vi "Periodic Tasks.vi"(8 "error in":errorcluster) -> ()   [LabVIEW 2017]
doc: "This VI runs in parallel to other tasks. It can contain as many user-defined periodic loops as you need. These can carry out PID or other sorts of timed response."
uses:
  <vilib>/Rock Robotics/WPI/Solenoid/WPI_SolenoidValue.ctl
  <vilib>/Rock Robotics/WPI/ThirdParty/Phoenix-LabVIEW/Motor Controller/Controls/CTRE_Phoenix_MotorControl_ControlMode.ctl
  <vilib>/Rock Robotics/WPI/DriverStation/WPI_DriverStationRobotMode2.ctl
  LabVIEW_is_Under_Control.lib/Util/Toggle/Change Detect.vi
  LabVIEW_is_Under_Control.lib/Util/Toggle/Change Detect Boolean.vi
  Robot Global Data.vi
  <vilib>/Rock Robotics/WPI/Solenoid/WPI_SolenoidSetEnum.vi
panel:
  out "Yaw":dbl
  in  "Exchange":dbl
  in  "ScoringHigh":dbl
  in  "Scoring Low":dbl
  in  "Reset":bool
  in  "Gains Elevador":T1={"proportional gain (Kc)"=1.0, "integral time (Ti, min)"=0.01, "derivative time (Td, min)"=0.0} {"derivative time (Td, min)" format="%.3f"; "integral time (Ti, min)" format="%.3f"; "proportional gain (Kc)" format="%.3f"}
  in  "Range Elevador":cluster{"output high":dbl, "output low":dbl}={"output high"=0.6, "output low"=-0.6} {"output low" format="%.2f"; "output high" format="%.2f"}
  in  "Enable squared":bool
  in  "Score":dbl=-0.3
  in  "Segurando":dbl=0.3
  in  "Expelir":dbl=-0.3
  in  "Coletar":dbl=0.9
  # "Intake"
  # "Drivetrain"
  # "Elevador"
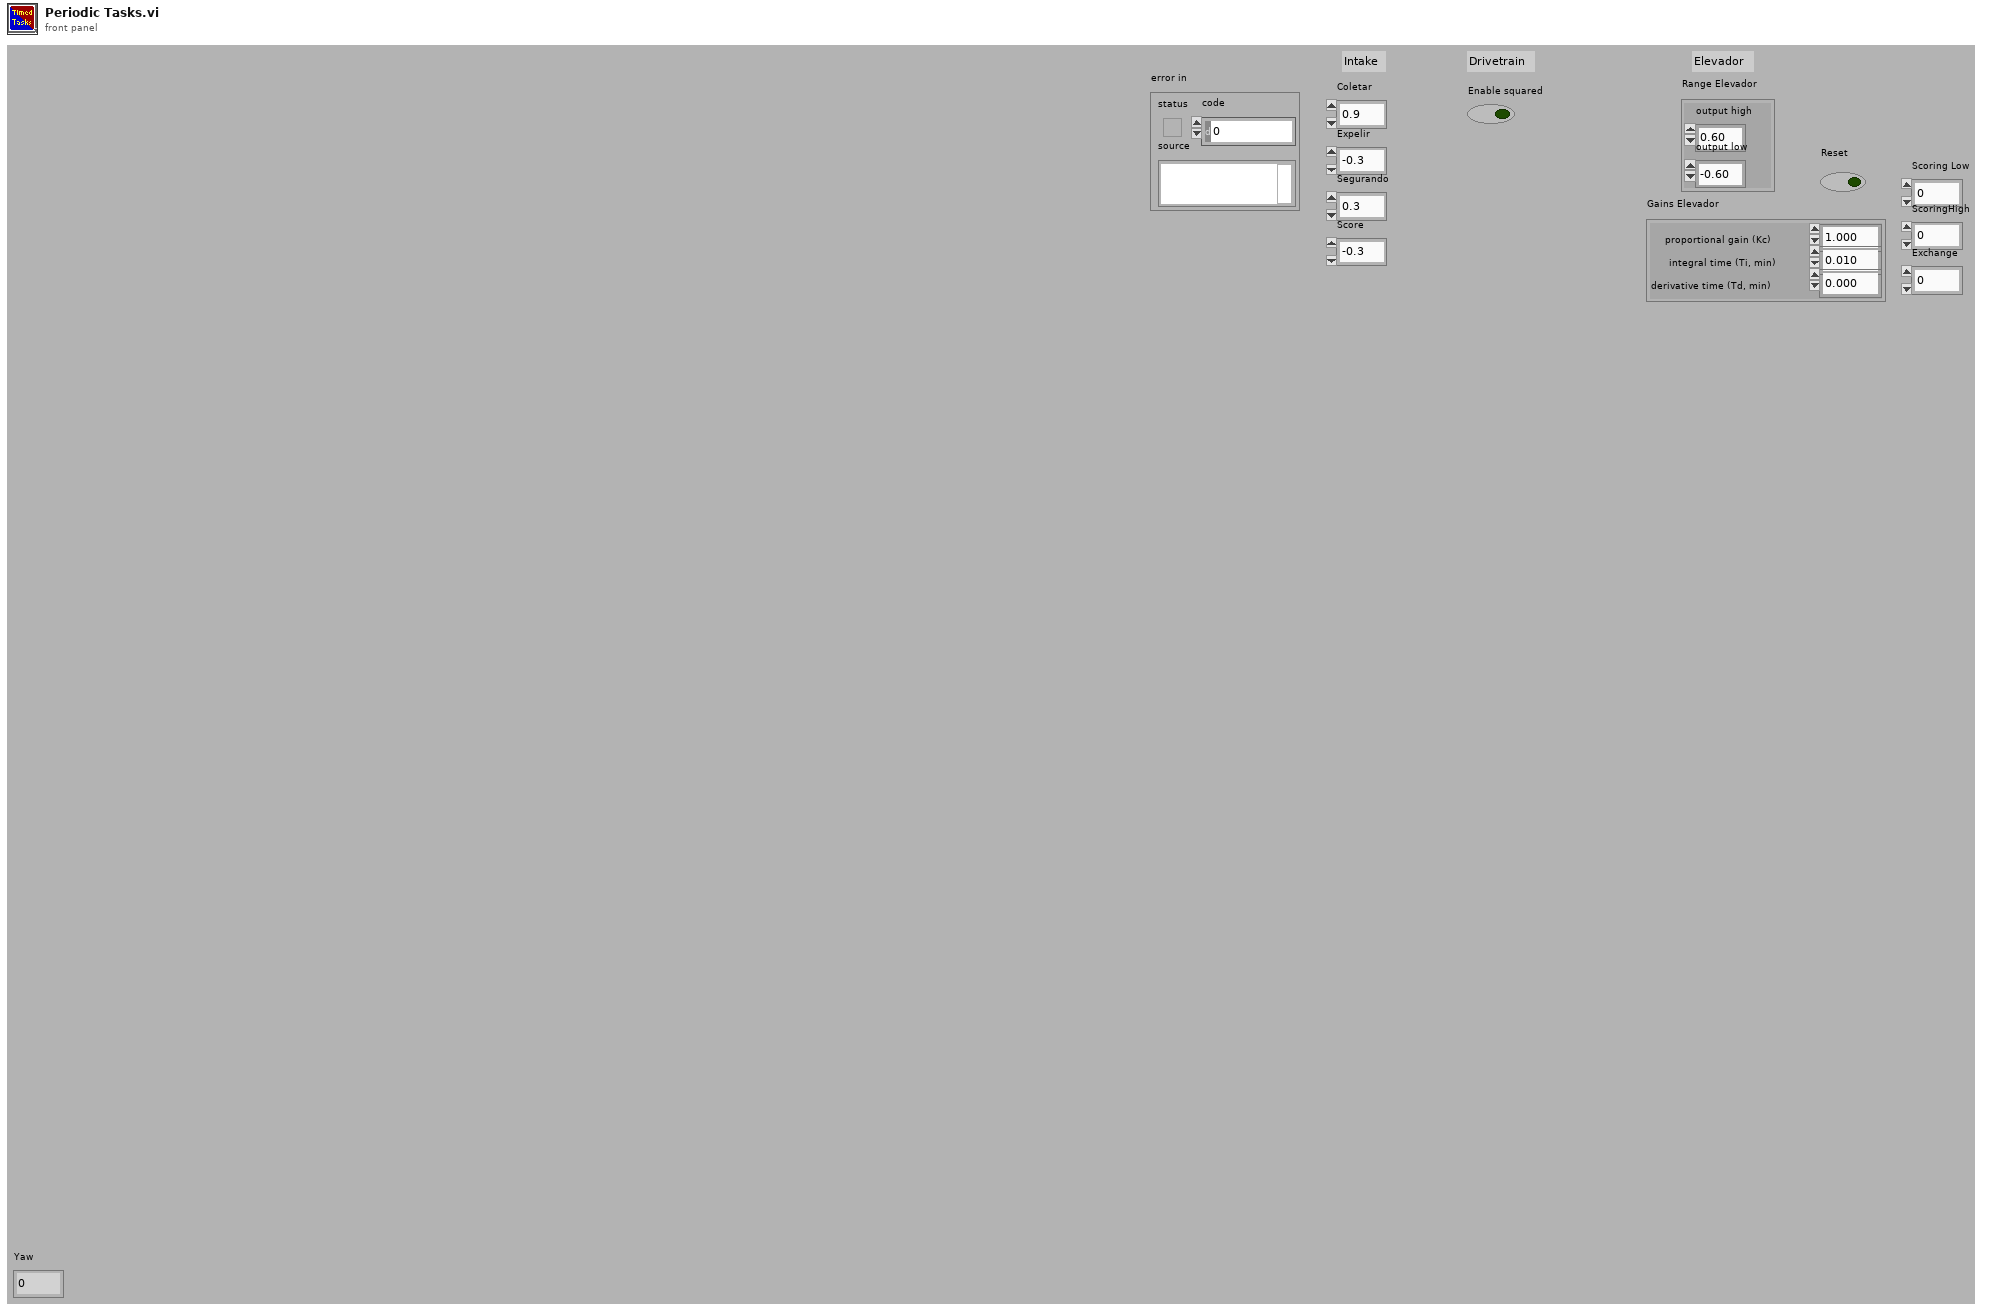
[diagram p1: front panel]
types:
  T1 = cluster{"proportional gain (Kc)":dbl, "integral time (Ti, min)":dbl, "derivative time (Td, min)":dbl}
  T2 = typedef "Máquina de estado do elevador.ctl" = enum16{"Resting", "Scoring Low", "Scoring Higher", "Exchange"}
  T3 = enum16{"Repouso", "Coletando", "Segurando", "Score"}
  T4 = typedef "WPI_SwitchDevRef.ctl" = cluster{"DevStatus":errorcluster, "DIO Channel":T5, "CntIndex":T6, "Normally Closed":bool}
  T5 = typedef "FPGA_DIOChannel.ctl" = enum8{"DIO 0", "DIO 1", "DIO 2", "DIO 3", "DIO 4", "DIO 5", "DIO 6", "DIO 7", "DIO 8", "DIO 9", "DIO MXP 0", "DIO MXP 1", "DIO MXP 2", "DIO MXP 3", "DIO MXP 4", "DIO MXP 5", "DIO MXP 6", "DIO MXP 7", "DIO MXP 8", "DIO MXP 9", "DIO MXP 10", "DIO MXP 11", "DIO MXP 12", "DIO MXP 13", "DIO MXP 14", "DIO MXP 15", "SPI Port CS1", "SPI Port CS2", "SPI Port CS3", "SPI Port MISO", "SPI Port MOSI", "Invalid"}
  T6 = typedef "FPGA_CounterCtrSystemIndex.ctl" = enum8{"Ctr 0", "Ctr 1", "Ctr 2", "Ctr 3", "Ctr 4", "Ctr 5", "Ctr 6", "Ctr 7", "Invalid"}
  T7 = typedef "WPI_EncoderDevRef.ctl" = cluster{"DevStatus":errorcluster, "EncoderIndex":T8, "CounterIndex":T6, "DistancePerCount":dbl, "Decoding Type":T9}
  T8 = typedef "FPGA_EncoderIdx.ctl" = enum8{"Enc 0", "Enc 1", "Enc 2", "Enc 3", "Enc 4", "Enc 5", "Enc 6", "Enc 7", "Invalid"}
  T9 = typedef "WPI_EncoderType.ctl" = enum16{"1x", "2x", "4x"}
  T10 = typedef "WPI_SolenoidDevRef.ctl" = cluster{"DevStatus":errorcluster, "Pneumatics Control Module":u8, "Forward Solenoid Channel":T11, "Reverse Solenoid Channel":T11}
  T11 = typedef "WPI_SolenoidChannel.ctl" = enum8{"Solenoid 0", "Solenoid 1", "Solenoid 2", "Solenoid 3", "Solenoid 4", "Solenoid 5", "Solenoid 6", "Solenoid 7", "Invalid"}
  T12 = typedef "WPI_MotorControlDeviceRef.ctl" = cluster{"DeviceStatus":errorcluster, "Type":T13, "PWM":cluster{"PWM Channel":T14, "DeadBand":T15}, "CAN":cluster{"Device Number":u8, "SetOutput VI Ref":variant, "GetOutput VI Ref":variant, "Enable VI Ref":variant, "Disable VI Ref":variant, "Data":variant}, "Invert":bool, "DIO PWM":cluster{"PWM \"Enable\" Channel":T14, "DIOChannel":T5, "PWM Rate":dbl}}
  T13 = typedef "WPI_MotorControlType.ctl" = enum16{"PWM", "CAN", "DIO PWM"}
  T14 = typedef "FPGA_DIOPWMChannel.ctl" = enum8{"PWM 0", "PWM 1", "PWM 2", "PWM 3", "PWM 4", "PWM 5", "PWM 6", "PWM 7", "PWM 8", "PWM 9", "PWM MXP 0", "PWM MXP 1", "PWM MXP 2", "PWM MXP 3", "PWM MXP 4", "PWM MXP 5", "PWM MXP 6", "PWM MXP 7", "PWM MXP 8", "PWM MXP 9", "Invalid"}
  T15 = typedef "WPI_PWMDeadband.ctl" = cluster{"Name":string, "maxPositivePwm":i32, "minPositivePwm":i32, "centerPwm":i32, "maxNegativePwm":i32, "minNegativePwm":i32, "angularRange":u16}
  T16 = cluster{"Yaw":dbl, "Roll":dbl, "Pitch":dbl, "Heading":dbl, "Fused Heading":dbl}
  T17 = typedef "WPI_SolenoidValue.ctl" = enum16{"Off", "On", "Forward", "Reverse"}
  T18 = typedef "WPI_DriverStationRobotMode2.ctl" = enum16{"Autonomous Disabled", "Autonomous Enabled", "Teleop Disabled", "Teleop Enabled", "Disconnected", "Finish", "Test Disabled", "Test Enabled", "Emergency Stopped"}
  T19 = typedef "CTRE_Phoenix_MotorControl_ControlMode.ctl" = u16
  T20 = typedef "Axes Cluster.ctl" = cluster{"Axes[0]":dbl, "Axes[1]":dbl, "Axes[2]":dbl, "Axes[3]":dbl, "Axes[4]":dbl, "Axes[5]":dbl, "Axes[6]":dbl, "Axes[7]":dbl, "Axes[8]":dbl}
  T21 = typedef "Button Cluster.ctl" = cluster{"Buttons[0]":bool, "Buttons[1]":bool, "Buttons[2]":bool, "Buttons[3]":bool, "Buttons[4]":bool, "Buttons[5]":bool, "Buttons[6]":bool, "Buttons[7]":bool, "Buttons[8]":bool, "Buttons[9]":bool}
  T22 = typedef "D-Pad.ctl" = cluster{"Top":bool, "Bottom":bool, "None":bool, "Right":bool, "Left":bool}
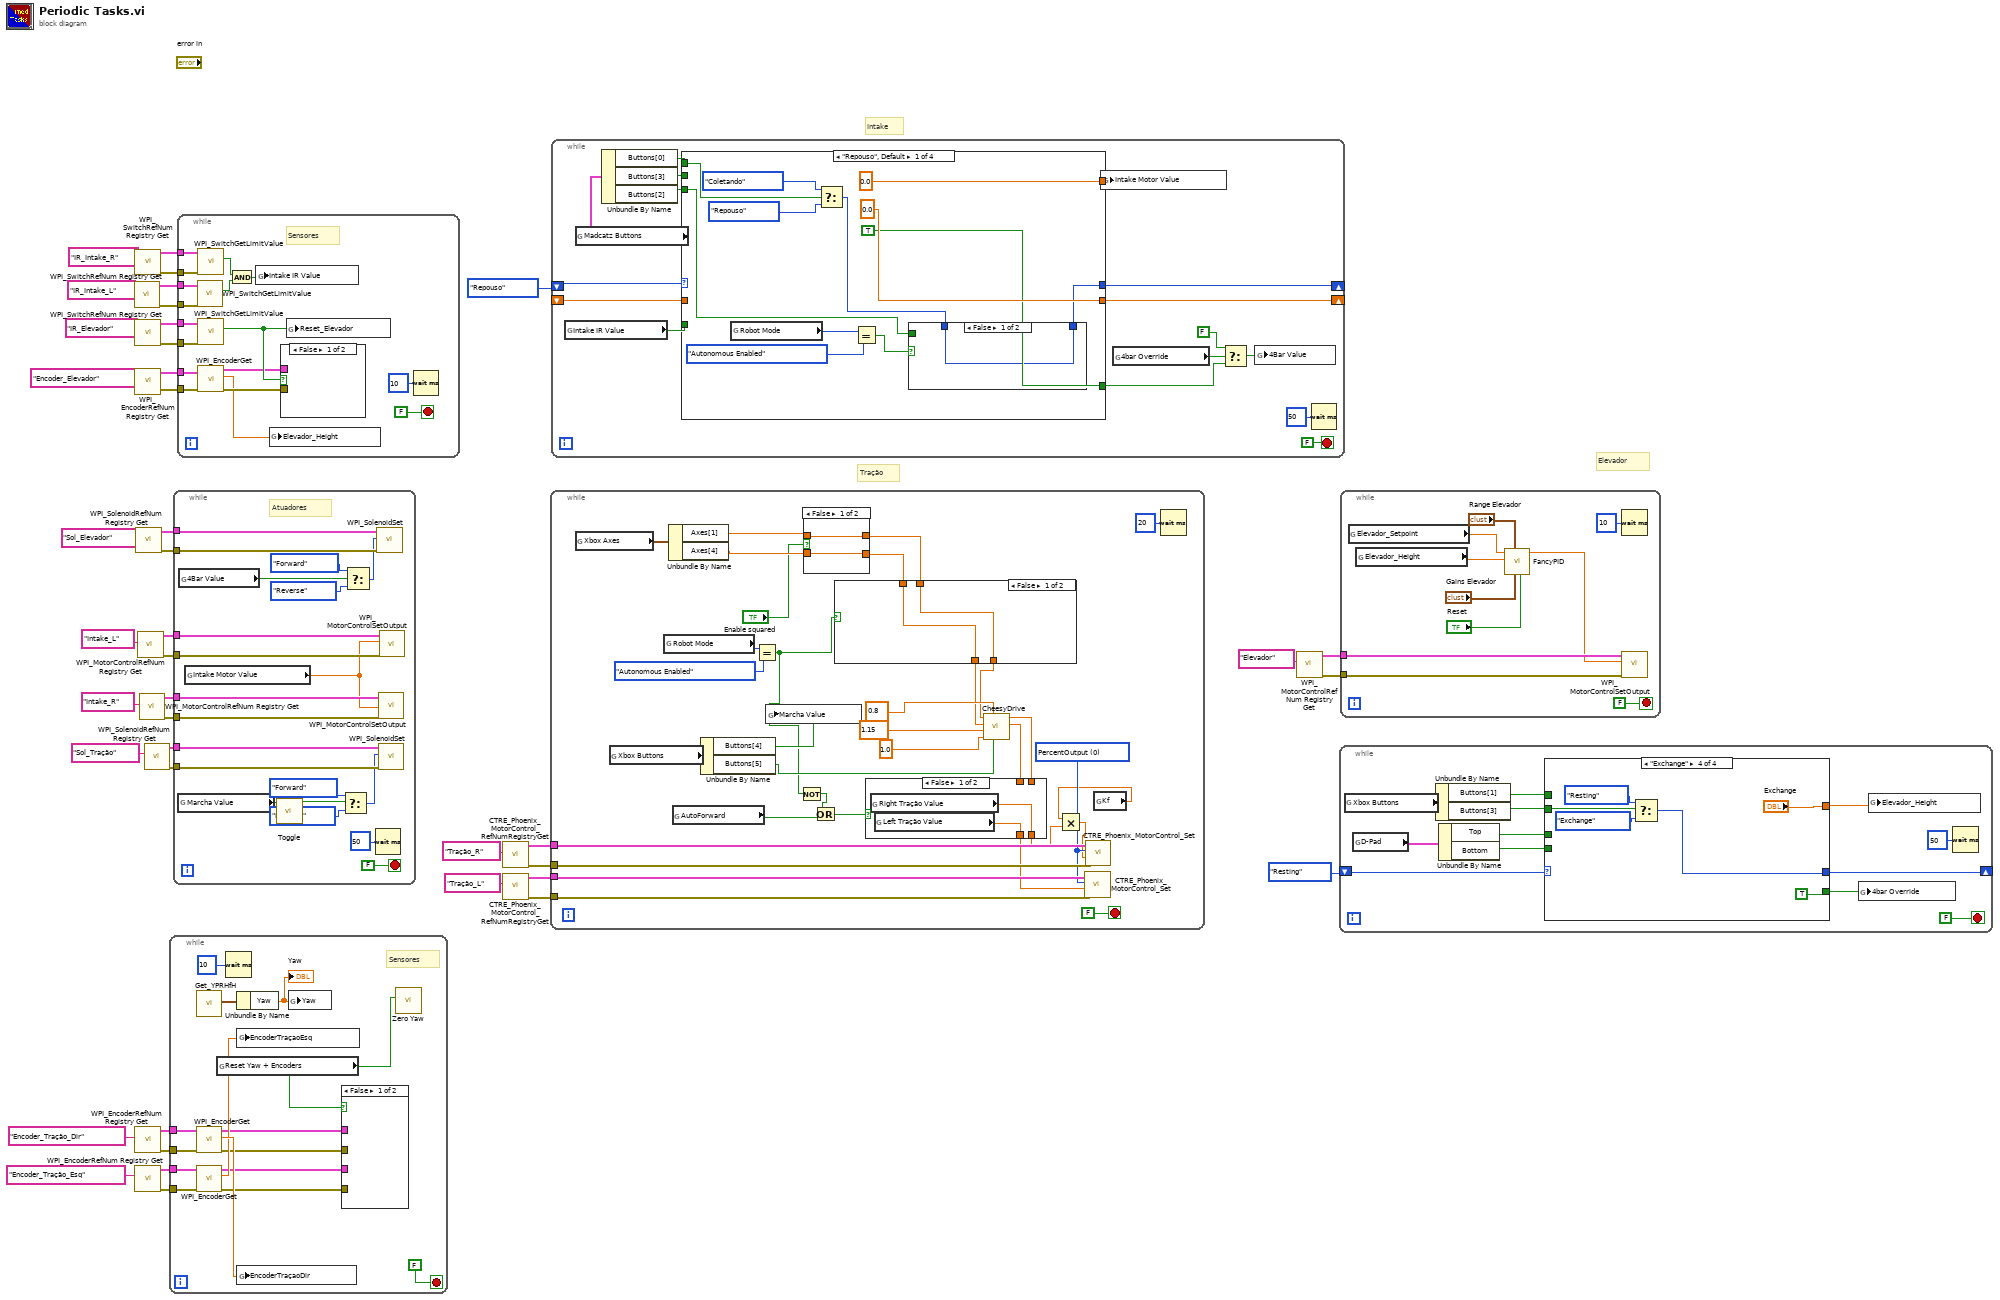
[diagram p0: block diagram]
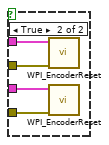
[diagram p2: hidden frame]
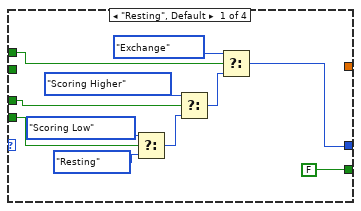
[diagram p3: hidden frame]
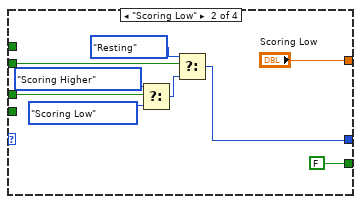
[diagram p4: hidden frame]
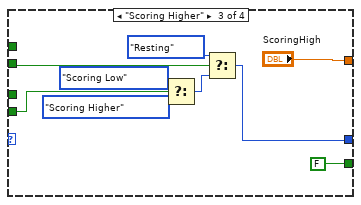
[diagram p5: hidden frame]
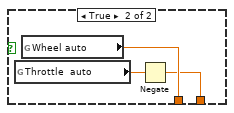
[diagram p7: hidden frame]
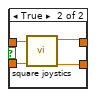
[diagram p8: hidden frame]
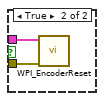
[diagram p9: hidden frame]
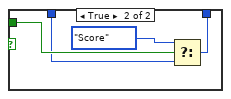
[diagram p10: hidden frame]
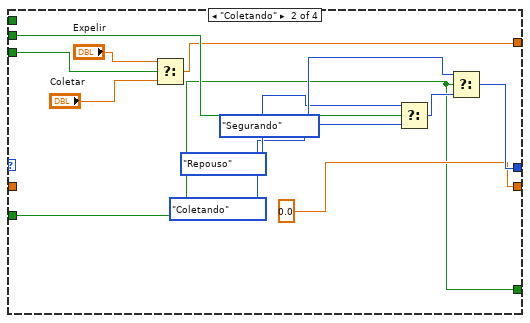
[diagram p11: hidden frame]
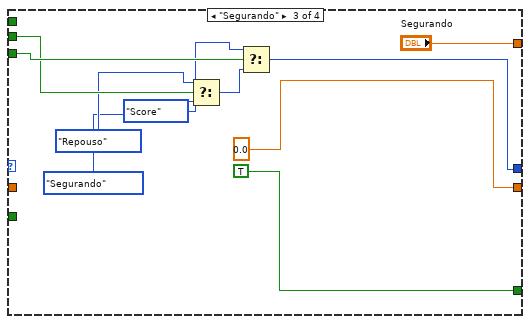
[diagram p12: hidden frame]
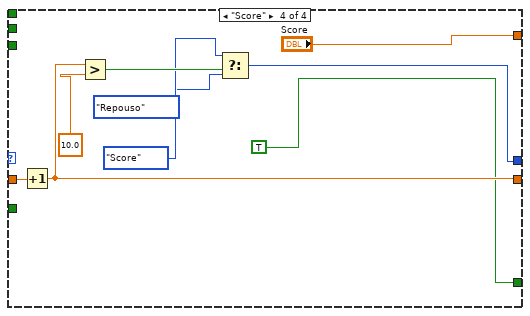
[diagram p13: hidden frame]
diagram:
  # "Elevador"
  # "Tração"
  # "Intake"
  n1 = call <vilib>:"WPI_SwitchRefNum Registry Get.vi"("refnum name"="IR_Intake_L") -> ("error out"=w38:errorcluster, "SwitchDevRef"=w37:T4)  [unwired: 9 in]
  n2 = call <vilib>:"WPI_SwitchRefNum Registry Get.vi"("refnum name"="IR_Intake_R") -> ("error out"=w36:errorcluster, "SwitchDevRef"=w35:T4)  [unwired: 9 in]
  n3 = call <vilib>:"WPI_SwitchRefNum Registry Get.vi"("refnum name"="IR_Elevador") -> ("error out"=w15:errorcluster, "SwitchDevRef"=w16:T4)  [unwired: 9 in]
  n4 = call <vilib>:"WPI_EncoderRefNum Registry Get.vi"("refnum name"="Encoder_Elevador") -> ("error out"=w11:errorcluster, "EncoderDevRef"=w12:T7)  [unwired: 9 in]
  n5 = call <vilib>:"WPI_EncoderRefNum Registry Get.vi"("refnum name"="Encoder_Tração_Dir") -> ("error out"=w4:errorcluster, "EncoderDevRef"=w5:T7)  [unwired: 9 in]
  n6 = call <vilib>:"WPI_EncoderRefNum Registry Get.vi"("refnum name"="Encoder_Tração_Esq") -> ("error out"=w3:errorcluster, "EncoderDevRef"=w2:T7)  [unwired: 9 in]
  n7 = call <vilib>:"WPI_SolenoidRefNum Registry Get.vi"("refnum name"="Sol_Elevador") -> ("error out"=w33:errorcluster, "SolenoidDevRef"=w32:T10)  [unwired: 9 in]
  n8 = call <vilib>:"WPI_MotorControlRefNum Registry Get.vi"("refnum name"="Intake_L") -> ("error out"=w31:errorcluster, "MotorControlDevRef"=w30:T12)  [unwired: 9 in]
  n9 = call <vilib>:"WPI_MotorControlRefNum Registry Get.vi"("refnum name"="Intake_R") -> ("error out"=w26:errorcluster, "MotorControlDevRef"=w27:T12)  [unwired: 9 in]
  n10 = call <vilib>:"WPI_SolenoidRefNum Registry Get.vi"("refnum name"="Sol_Tração") -> ("error out"=w23:errorcluster, "SolenoidDevRef"=w24:T10)  [unwired: 9 in]
  n11 = while {
    tunnel: w5 -> [w56]
    tunnel: w4 -> [w55]
    tunnel: w2 -> [w51]
    tunnel: w3 -> [w52]
    stop <- FALSE stop-if-true
    # "Sensores"
    n12 = call <vilib>:"Get_YPRHfH.vi"() -> ("YRPHfH"=w44:T16)  [unwired: 11 in]
    n13 = call <vilib>:"WPI_EncoderGet.vi"("error in (no error)"=w55, "EncoderDevRef"=w56) -> ("error out"=w47:errorcluster, "Distance"=w54:dbl, "EncoderDevRef"=w48:T7)  [unwired: 4 in, 3 out]
    n14 = call <vilib>:"WPI_EncoderGet.vi"("error in (no error)"=w52, "EncoderDevRef"=w51) -> ("error out"=w45:errorcluster, "Distance"=w53:dbl, "EncoderDevRef"=w46:T7)  [unwired: 4 in, 3 out]
    n15 = global read "Robot Global Data.vi" "Reset Yaw + Encoders"() -> (w42:bool)
    n16 = Wait (ms)(milliseconds to wait=u32 10) -> ()  [unwired: 1 out]
    n17 = Unbundle By Name(w44) -> ("Yaw"=w43:dbl)
    "Yaw" <- w43
    n18 = global write "Robot Global Data.vi" "EncoderTraçaoEsq"(w53) -> ()
    n19 = global write "Robot Global Data.vi" "EncoderTraçaoDir"(w54) -> ()
    n20 = global write "Robot Global Data.vi" "Yaw"(w43) -> ()
    n21 = case shown="False" w42 {
      tunnel: w48 -> [_ w60]
      tunnel: w47 -> [_ w59]
      tunnel: w46 -> [_ w58]
      tunnel: w45 -> [_ w57]
      frame False {
      }
      frame True {
        n22 = call <vilib>:"WPI_EncoderReset.vi"("error in (no error)"=w59, "EncoderDevRef"=w60) -> ()  [unwired: 8 in, 2 out]
        n23 = call <vilib>:"WPI_EncoderReset.vi"("error in (no error)"=w57, "EncoderDevRef"=w58) -> ()  [unwired: 8 in, 2 out]
      }
    }
    n24 = call <vilib>:"Zero Yaw.vi"("Zero"=w42) -> ()  [unwired: 11 in]
  }
  n25 = while {
    tunnel: w33 -> [w80]
    tunnel: w32 -> [w79]
    tunnel: w31 -> [w74]
    tunnel: w30 -> [w73]
    tunnel: w27 -> [w72]
    tunnel: w26 -> [w71]
    tunnel: w24 -> [w65]
    tunnel: w23 -> [w64]
    stop <- FALSE stop-if-true
    # "Atuadores"
    n26 = global read "Robot Global Data.vi" "Marcha Value"() -> (w62:bool)
    n27 = global read "Robot Global Data.vi" "4Bar Value"() -> (w75:bool)
    n28 = global read "Robot Global Data.vi" "Intake Motor Value"() -> (w70:dbl)
    n29 = call "Toggle.vi"("In"=w62) -> ("Toggled"=w61:bool)  [unwired: 10 in]
    n30 = Select(t=WPI_SolenoidValue."Forward" ("Value"), s=w61, f=WPI_SolenoidValue."Reverse" ("Value")) -> (s? t:f=w63:T17)
    n31 = Select(t=WPI_SolenoidValue."Forward" ("Value"), s=w75, f=WPI_SolenoidValue."Reverse" ("Value")) -> (s? t:f=w78:T17)
    n32 = Wait (ms)(milliseconds to wait=u32 50) -> ()  [unwired: 1 out]
    n33 = call-poly <vilib>:"WPI_SolenoidSet.vi"("error in (no error)"=w80, "Value"=w78, "SolenoidDevRef"=w79) -> ()  [unwired: 7 in, 2 out]
    n34 = call <vilib>:"WPI_MotorControlSetOutput.vi"("error in (no error)"=w71, "Output"=w70, "MotorControlDevRef"=w72) -> ()  [unwired: 6 in, 3 out]
    n35 = call-poly <vilib>:"WPI_SolenoidSet.vi"("error in (no error)"=w64, "Value"=w63, "SolenoidDevRef"=w65) -> ()  [unwired: 7 in, 2 out]
    n36 = call <vilib>:"WPI_MotorControlSetOutput.vi"("error in (no error)"=w74, "Output"=w70, "MotorControlDevRef"=w73) -> ()  [unwired: 6 in, 3 out]
  }
  n37 = while {
    tunnel: w38 -> [w92]
    tunnel: w37 -> [w91]
    tunnel: w36 -> [w90]
    tunnel: w35 -> [w89]
    tunnel: w15 -> [w87]
    tunnel: w16 -> [w88]
    tunnel: w12 -> [w86]
    tunnel: w11 -> [w85]
    stop <- FALSE stop-if-true
    # "Sensores"
    n38 = call <vilib>:"WPI_SwitchGetLimitValue.vi"("error in (no error)"=w92, "SwitchDevRef"=w91) -> ("Switch Pressed"=w97:bool)  [unwired: 7 in, 2 out]
    n39 = call <vilib>:"WPI_SwitchGetLimitValue.vi"("error in (no error)"=w90, "SwitchDevRef"=w89) -> ("Switch Pressed"=w96:bool)  [unwired: 7 in, 2 out]
    n40 = call <vilib>:"WPI_SwitchGetLimitValue.vi"("error in (no error)"=w87, "SwitchDevRef"=w88) -> ("Switch Pressed"=w84:bool)  [unwired: 7 in, 2 out]
    n41 = call <vilib>:"WPI_EncoderGet.vi"("error in (no error)"=w85, "EncoderDevRef"=w86) -> ("error out"=w82:errorcluster, "Distance"=w81:dbl, "EncoderDevRef"=w83:T7)  [unwired: 4 in, 3 out]
    n42 = And(x=w96, y=w97) -> (x .and. y?=w93:bool)
    n43 = global write "Robot Global Data.vi" "Intake IR Value"(w93) -> ()
    n44 = global write "Robot Global Data.vi" "Elevador_Height"(w81) -> ()
    n45 = case shown="False" w84 {
      tunnel: w83 -> [_ w99]
      tunnel: w82 -> [_ w98]
      frame False {
      }
      frame True {
        n46 = call <vilib>:"WPI_EncoderReset.vi"("error in (no error)"=w98, "EncoderDevRef"=w99) -> ()  [unwired: 8 in, 2 out]
      }
    }
    n47 = global write "Robot Global Data.vi" "Reset_Elevador"(w84) -> ()
    n48 = Wait (ms)(milliseconds to wait=u32 10) -> ()  [unwired: 1 out]
  }
  n49 = call <vilib>:"CTRE_Phoenix_MotorControl_RefNumRegistryGet.vi"("refnum name"="Tração_R") -> ("error out"=w18:errorcluster, "PhoenixMotorControlDevRef"=w20:T12)  [unwired: 9 in]
  n50 = call <vilib>:"CTRE_Phoenix_MotorControl_RefNumRegistryGet.vi"("refnum name"="Tração_L") -> ("error out"=w17:errorcluster, "PhoenixMotorControlDevRef"=w19:T12)  [unwired: 9 in]
  n51 = while {
    tunnel: w20 -> [w123]
    tunnel: w19 -> [w122]
    tunnel: w18 -> [w121]
    tunnel: w17 -> [w120]
    stop <- FALSE stop-if-true
    w119 = T19 0 items=["PercentOutput"=0, "Position"=1, "Velocity"=2, "Current"=3, "Follower"=5, "MotionProfile"=6, "MotionMagic"=7, "MotionMagicArc"=8, "MotionProfileArc"=10, "Disabled"=15] ("Control Mode")
    n52 = global read "Robot Global Data.vi" "Xbox Axes"() -> (w132:T20)
    n53 = global read "Robot Global Data.vi" "Xbox Buttons"() -> (w130:T21)
    n54 = global read "Robot Global Data.vi" "Robot Mode"() -> (w115:T18)
    n55 = Unbundle By Name(w132) -> ("Axes[1]"=w117:dbl, "Axes[4]"=w118:dbl)
    n56 = global read "Robot Global Data.vi" "AutoForward"() -> (w104:bool)
    n57 = Unbundle By Name(w130) -> ("Buttons[4]"=w128:bool, "Buttons[5]"=w129:bool)
    n58 = Equal?(x=w115, y=WPI_DriverStationRobotMode2."Autonomous Enabled") -> (x = y?=w103:bool)
    n59 = global write "Robot Global Data.vi" "Marcha Value"(w128) -> ()
    n60 = Not(x=w103) -> (.not. x?=w106:bool)
    n61 = case shown="False" "Enable squared" {
      tunnel: w118 -> [w143 w147]
      tunnel: [w143 w146] -> w112
      tunnel: w117 -> [w142 w145]
      tunnel: [w142 w144] -> w113
      frame False {
      }
      frame True {
        n62 = call "square joystics.vi"("right joy"=w147, "left joy"=w145) -> ("Right Out"=w146:dbl, "Left Out"=w144:dbl)  [unwired: 8 in]
      }
    }
    n63 = Or(x=w106, y=w104) -> (x .or. y?=w105:bool)
    n64 = case shown="False" w103 {
      tunnel: [w137 w141] -> w107
      tunnel: [w138 w139] -> w108
      tunnel: w113 -> [w138 _]
      tunnel: w112 -> [w137 _]
      frame False {
      }
      frame True {
        n65 = global read "Robot Global Data.vi" "Throttle  auto"() -> (w140:dbl)
        n66 = global read "Robot Global Data.vi" "Wheel auto"() -> (w141:dbl)
        n67 = Negate(x=w140) -> (-x=w139:dbl)
      }
    }
    n68 = call "CheesyDrive.vi"("Quickturn"=w129, "WheelNonLinearity"=0.8, "negInertiaScalar"=1.0, "Sensitivty"=1.15, "Wheel"=w107, "Throttle"=w108) -> ("Right PWM"=w109:dbl, "Left PWM"=w111:dbl)  [unwired: 4 in]
    n69 = case shown="False" w105 {
      tunnel: [w133 w135] -> w102
      tunnel: w111 -> [_ w135]
      tunnel: [w134 w136] -> w110
      tunnel: w109 -> [_ w136]
      frame False {
        n70 = global read "Robot Global Data.vi" "Right Tração Value"() -> (w133:dbl)
        n71 = global read "Robot Global Data.vi" "Left Tração Value"() -> (w134:dbl)
      }
      frame True {
      }
    }
    n72 = call <vilib>:"CTRE_Phoenix_MotorControl_Set.vi"("error in (no error)"=w120, "Output"=w110, "Control Mode"=w119, "PhoenixMotorControlDevRef"=w122) -> ()  [unwired: 6 in, 2 out]
    n73 = global read "Robot Global Data.vi" "Kf"() -> (w101:dbl)
    n74 = Multiply(x=w101, y=w102) -> (x*y=w100:dbl)
    n75 = call <vilib>:"CTRE_Phoenix_MotorControl_Set.vi"("error in (no error)"=w121, "Output"=w100, "Control Mode"=w119, "PhoenixMotorControlDevRef"=w123) -> ()  [unwired: 6 in, 2 out]
    n76 = Wait (ms)(milliseconds to wait=u32 20) -> ()  [unwired: 1 out]
  }
  n77 = while {
    shift-right: [w159] -> _
    shift-left: T3."Repouso" -> [w163]
    shift-right: [w156] -> _
    shift-left: _ -> [w157]
    stop <- FALSE stop-if-true
    n78 = global read "Robot Global Data.vi" "Intake IR Value"() -> (w158:bool)
    n79 = global read "Robot Global Data.vi" "Madcatz Buttons"() -> (w160:T21)
    n80 = Unbundle By Name(w160) -> ("Buttons[0]"=w152:bool, "Buttons[3]"=w154:bool, "Buttons[2]"=w153:bool)
    n81 = case shown="\"Repouso\", Default" w163 {
      tunnel: w152 -> [w175 _ _ _]
      tunnel: [w165 w188 w196 w205] -> w159
      tunnel: w154 -> [_ w191 w200 _]
      tunnel: w158 -> [_ w182 _ _]
      tunnel: w153 -> [w164 w181 w202 _]
      tunnel: w157 -> [_ _ _ w211]
      tunnel: [0.0 0.0 0.0 w210] -> w156
      tunnel: [0.0 w183 "Segurando" "Score"] -> w155
      tunnel: [TRUE w182 TRUE TRUE] -> w150
      frame "Repouso", Default {
        n82 = global read "Robot Global Data.vi" "Robot Mode"() -> (w168:T18)
        n83 = Select(t=T3."Coletando", s=w175, f=T3."Repouso") -> (s? t:f=w166:T3)
        n84 = Equal?(x=w168, y=WPI_DriverStationRobotMode2."Autonomous Enabled") -> (x = y?=w167:bool)
        n85 = case shown="False" w167 {
          tunnel: w164 -> [_ w180]
          tunnel: w166 -> [w176 w179]
          tunnel: [w176 w177] -> w165
          frame False {
          }
          frame True {
            n86 = Select(t=T3."Score", s=w180, f=w179) -> (s? t:f=w177:T3)
          }
        }
      }
      frame "Coletando" {
        n87 = Select(t="Expelir", s=w181, f="Coletar") -> (s? t:f=w183:dbl)
        n88 = Select(t=T3."Repouso", s=w191, f=T3."Coletando") -> (s? t:f=w185:T3)
        n89 = Select(t=T3."Segurando", s=w182, f=w185) -> (s? t:f=w188:T3)
      }
      frame "Segurando" {
        n90 = Select(t=T3."Repouso", s=w200, f=T3."Segurando") -> (s? t:f=w199:T3)
        n91 = Select(t=T3."Score", s=w202, f=w199) -> (s? t:f=w196:T3)
      }
      frame "Score" {
        n92 = Increment(x=w211) -> (x+1=w210:dbl)
        n93 = Greater?(x=w210, y=10.0) -> (0:w208:bool)
        n94 = Select(t=T3."Repouso", s=w208, f=T3."Score") -> (s? t:f=w205:T3)
      }
    }
    n95 = global write "Robot Global Data.vi" "Intake Motor Value"(w155) -> ()
    n96 = global read "Robot Global Data.vi" "4bar Override"() -> (w151:bool)
    n97 = Select(t=FALSE, s=w151, f=w150) -> (s? t:f=w148:bool)
    n98 = global write "Robot Global Data.vi" "4Bar Value"(w148) -> ()
    n99 = Wait (ms)(milliseconds to wait=u32 50) -> ()  [unwired: 1 out]
  }
  n100 = call <vilib>:"WPI_MotorControlRefNum Registry Get.vi"("refnum name"="Elevador") -> ("error out"=w8:errorcluster, "MotorControlDevRef"=w9:T12)  [unwired: 9 in]
  n101 = while {
    shift-right: [w213] -> _
    shift-left: Máquina_de_estado_do_elevador."Resting" -> [w214]
    stop <- FALSE stop-if-true
    n102 = global read "Robot Global Data.vi" "Xbox Buttons"() -> (w220:T21)
    n103 = global read "Robot Global Data.vi" "D-Pad"() -> (w221:T22)
    n104 = Unbundle By Name(w220) -> ("Buttons[1]"=w215:bool, "Buttons[3]"=w219:bool)
    n105 = Unbundle By Name(w221) -> ("Top"=w218:bool, "Bottom"=w217:bool)
    n106 = case shown="\"Exchange\"" w214 {
      tunnel: w219 -> [_ w242 w251 w257]
      tunnel: w218 -> [w233 w241 _ _]
      tunnel: w217 -> [w232 _ w249 _]
      tunnel: [_ "Scoring Low" "ScoringHigh" "Exchange"] -> w216
      tunnel: [w225 w239 w248 w256] -> w213
      tunnel: w215 -> [w230 _ _ _]
      tunnel: [FALSE FALSE FALSE TRUE] -> w212
      frame "Resting", Default {
        n107 = Select(t=Máquina_de_estado_do_elevador."Scoring Low", s=w232, f=Máquina_de_estado_do_elevador."Resting") -> (s? t:f=w234:T2)
        n108 = Select(t=Máquina_de_estado_do_elevador."Scoring Higher", s=w233, f=w234) -> (s? t:f=w231:T2)
        n109 = Select(t=Máquina_de_estado_do_elevador."Exchange", s=w230, f=w231) -> (s? t:f=w225:T2)
      }
      frame "Scoring Low" {
        n110 = Select(t=Máquina_de_estado_do_elevador."Scoring Higher", s=w241, f=Máquina_de_estado_do_elevador."Scoring Low") -> (s? t:f=w240:T2)
        n111 = Select(t=Máquina_de_estado_do_elevador."Resting", s=w242, f=w240) -> (s? t:f=w239:T2)
      }
      frame "Scoring Higher" {
        n112 = Select(t=Máquina_de_estado_do_elevador."Scoring Low", s=w249, f=Máquina_de_estado_do_elevador."Scoring Higher") -> (s? t:f=w250:T2)
        n113 = Select(t=Máquina_de_estado_do_elevador."Resting", s=w251, f=w250) -> (s? t:f=w248:T2)
      }
      frame "Exchange" {
        n114 = Select(t=Máquina_de_estado_do_elevador."Resting", s=w257, f=Máquina_de_estado_do_elevador."Exchange") -> (s? t:f=w256:T2)
      }
    }
    n115 = global write "Robot Global Data.vi" "4bar Override"(w212) -> ()
    n116 = global write "Robot Global Data.vi" "Elevador_Height"(w216) -> ()
    n117 = Wait (ms)(milliseconds to wait=u32 50) -> ()  [unwired: 1 out]
  }
  n118 = while {
    tunnel: w9 -> [w266]
    tunnel: w8 -> [w265]
    stop <- FALSE stop-if-true
    n119 = global read "Robot Global Data.vi" "Elevador_Setpoint"() -> (w260:dbl)
    n120 = global read "Robot Global Data.vi" "Elevador_Height"() -> (w259:dbl)
    n121 = call "FancyPID.vi"("Reset"="Reset", "Gains"="Gains Elevador", "Range"="Range Elevador", "Process variable"=w259, "Setpoint"=w260) -> ("output"=w264:dbl)  [unwired: 6 in]
    n122 = Wait (ms)(milliseconds to wait=u32 10) -> ()  [unwired: 1 out]
    n123 = call <vilib>:"WPI_MotorControlSetOutput.vi"("error in (no error)"=w265, "Output"=w264, "MotorControlDevRef"=w266) -> ()  [unwired: 6 in, 3 out]
  }
